vi "test start Julia & execute a REPL line.vi"() -> (0 "error out":errorcluster, 3 "return code":i32)   [LabVIEW 2018]
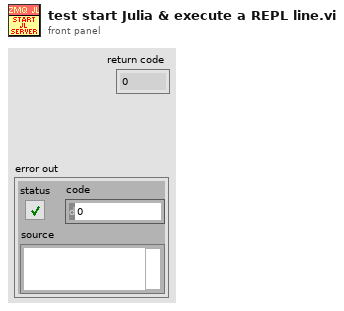
[diagram p1: front panel]
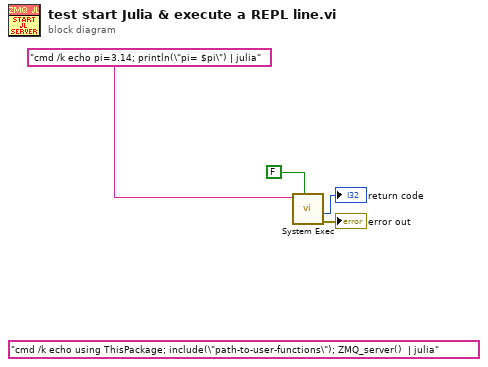
[diagram p0: block diagram]
diagram:
  (unwired) "cmd /k echo using ThisPackage; include(\"path-to-user-functions\"); ZMQ_server()  | julia"
  n1 = call <vilib>:"System Exec.vi"("wait until completion? (T)"=FALSE, "command line"="cmd /k echo pi=3.14; println(\"pi= $pi\") | julia") -> ("error out"=→"error out":errorcluster, "return code"=→"return code":i32)  [unwired: 6 in, 2 out]
